vi "Get Format.vi"(8 "error in":errorcluster, 11 "Formatter in":refnum<class "Formatter.lvclass">) -> (0 "error out":errorcluster, 2 "Format":string="%s - %-7s - %s - %s - %d - %s\\n", 3 "Formatter out":refnum<class "Formatter.lvclass">)   [LabVIEW 2016, in "hse-logger.lvlib" / "Formatter.lvclass"]
uses:
  Formatter.lvclass
  Formatter.lvclass/Formatter.ctl
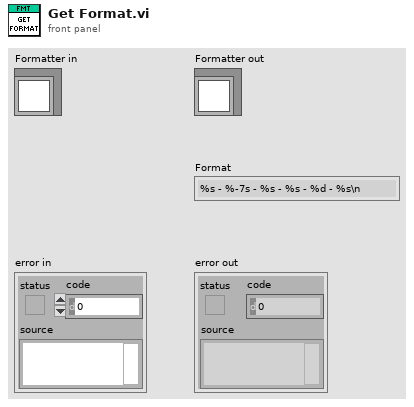
[diagram p1: front panel]
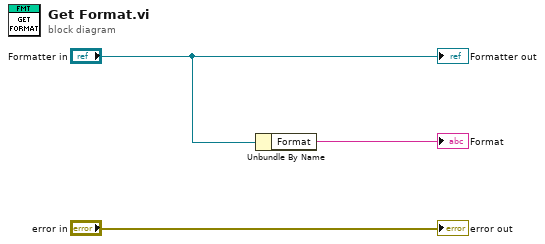
[diagram p0: block diagram]
diagram:
  n1 = Unbundle By Name("Formatter in") -> ("Format"=→"Format":string)
  "error out" <- "error in"
  "Formatter out" <- "Formatter in"
